vi "Actor Core.vi"(8 "error in":errorcluster, 11 "Elevator Controller in":refnum<class "Sim User Console Actor.lvclass">) -> (0 "error out":errorcluster, 3 "Actor out":refnum<class "Actor.lvclass">)   [LabVIEW 2019, in "Simulated User Console Actor.lvlib" / "Sim User Console Actor.lvclass"]
doc: "(<B>Filename</B>: Actor Framework.lvlib:Actor.lvclass:Actor Core.vi)\n\nReceives messages to the actor, reacts to them, and initiates any error handling that may shut the actor down.\n\nDescendant classes may override this VI to append parallel tasks for the actor to complete while it handles messages. Overrides use the Call Parent Method node."
uses:
  Sim User Console Actor.lvclass
  <vilib>/ActorFramework/Stop Msg/Stop Msg.lvclass
  <vilib>/ActorFramework/Actor/Actor.lvclass
  User Console Actor/User Console Actor/User Console Actor.lvclass
  C:/Workspace/CLA/Elevator AF 2nd/User Console Actor/User Console Actor/User Console Actor.lvclass
  C:/Program Files (x86)/National Instruments/LabVIEW 2019/vi.lib/ActorFramework/Actor/Actor.lvclass
  Elevator Controller/Elevator Controller Actor Messages/Restart Timing Msg/Restart Timing Msg.lvclass
  Elevator Controller/Elevator Controller Actor Messages/Change timing to seconds Msg/Change timing to seconds Msg.lvclass
  Elevator Controller/Elevator Controller Actor Messages/Set State Msg/Set State Msg.lvclass
  Elevator Controller/Elevator Controller/State -Enum.ctl
  Elevator Controller/Elevator Controller/Elevator Controller Actor.lvclass
  Elevator Controller/Elevator Controller Actor Messages/Call Emergency Msg/Call Emergency Msg.lvclass
  Door Buttons.ctl
  Elevator Call.ctl
  Floor Selection.ctl
panel:
  in  "Emergency":bool
  in  "Floor Selection":T1
  in  "Elevator Call":T2
  in  "Door Buttons":T3
  # "[Covers: UI1]\n[Covers: UI2]\n[Covers: UI2A] \n[Covers: UI2A1] \n[Covers: UI2A2] \n[Covers: UI2B] \n[Covers: UI2B1] \n[Covers: UI2B2] \n[Covers: UI2C] \n[Covers: UI2C1] \n[Covers: UI2C2] \n[Covers: UI2C3] \n[Covers: UI2D] \n[Covers: UI2D1]"
  # "Fourth Floor"
  # "Third Floor"
  # "Second Floor"
  # "First Floor"
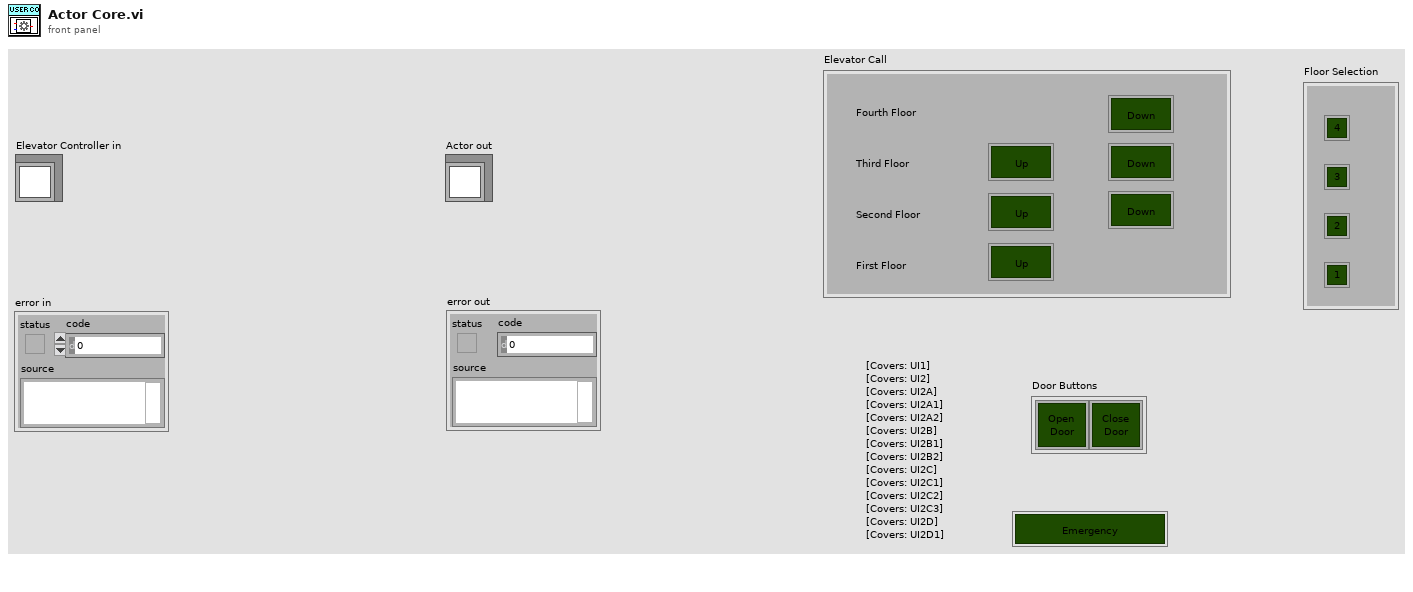
[diagram p1: front panel]
types:
  T1 = typedef "Simulated User Console Actor.lvlib/Sim User Console Actor.lvclass/Floor Selection.ctl" = cluster{"Floor4":bool, "Floor 3":bool, "Floor2":bool, "Floor1":bool}
  T2 = typedef "Simulated User Console Actor.lvlib/Sim User Console Actor.lvclass/Elevator Call.ctl" = cluster{"Up":bool, "Up 2":bool, "Up 3":bool, "Down":bool, "Down 2":bool, "Down 3":bool}
  T3 = typedef "Simulated User Console Actor.lvlib/Sim User Console Actor.lvclass/Door Buttons.ctl" = cluster{"Open Door":bool, "Close Door":bool}
  T4 = typedef "Elevator Controller Actor.lvlib/Elevator Controller Actor.lvclass/State -Enum.ctl" = enum16{"Initial", "Wait for First Request", "Start and Move", "Anaysis", "Continue Travel", "Stop at Floor", "Open and Close Door Sequence", "No Request Remaining", "Emergency Call", "Terminate Process"}
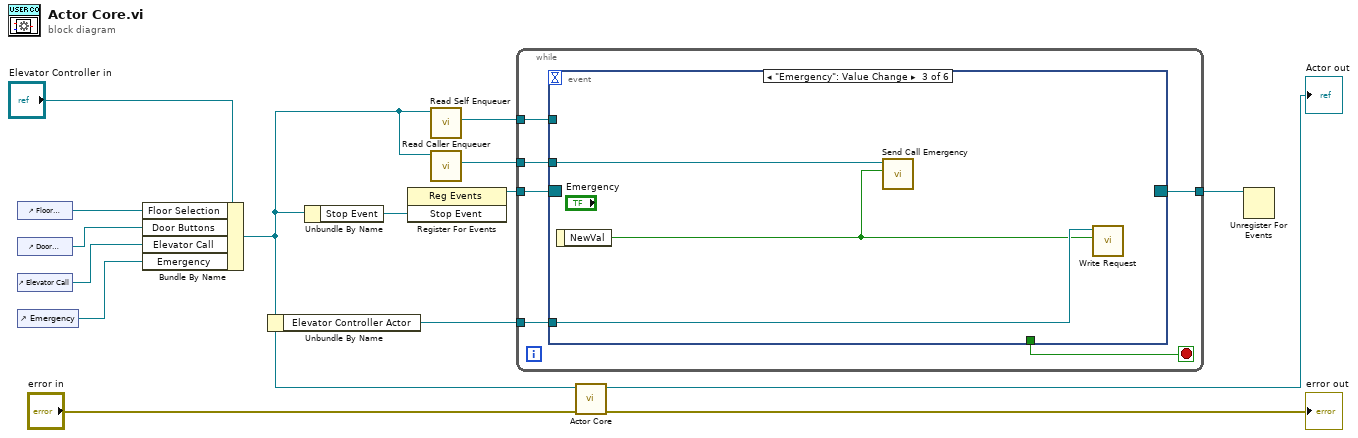
[diagram p0: block diagram]
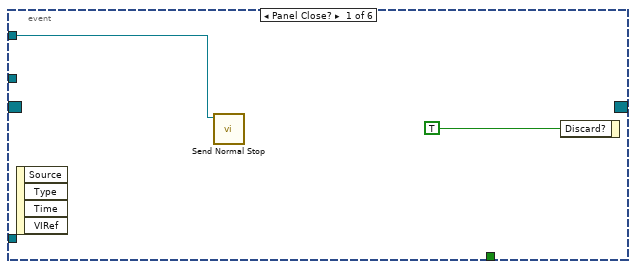
[diagram p2: hidden frame]
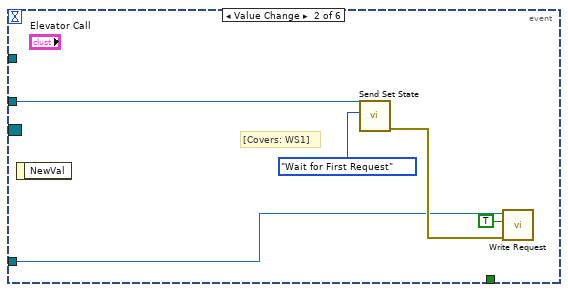
[diagram p3: hidden frame]
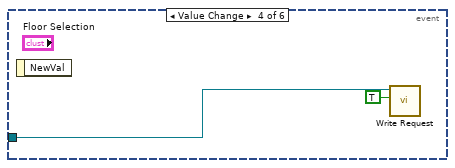
[diagram p4: hidden frame]
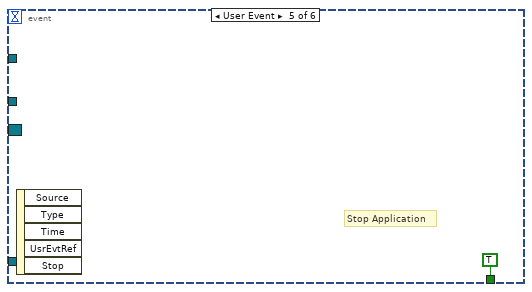
[diagram p5: hidden frame]
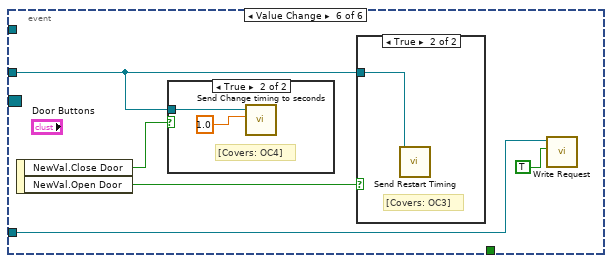
[diagram p6: hidden frame]
diagram:
  n1 = control-ref of="Floor Selection"() -> (w7:refnum<vi>)
  n2 = control-ref of="Door Buttons"() -> (w6:refnum<vi>)
  n3 = control-ref of="Elevator Call"() -> (w5:refnum<vi>)
  n4 = control-ref of="Emergency"() -> (w4:refnum<vi>)
  n5 = Bundle By Name(cluster="Elevator Controller in", "Floor Selection"=w7, "Door Buttons"=w6, "Elevator Call"=w5, "Emergency"=w4) -> (w2:refnum<class "Sim User Console Actor.lvclass">)
  n6 = Unbundle By Name(w2) -> ("Elevator Controller Actor"=w1:refnum<class "Elevator Controller Actor.lvclass">)
  n7 = Unbundle By Name(w2) -> ("Stop Event"=w12:refnum<user-event>)
  n8 = register-events(w12) -> (reference out=w11:refnum<event-registration>)  [unwired: 2 in, 1 out]
  n9 = call <vilib>:"Read Self Enqueuer.vi"("Actor"=w2) -> ("Self Enqueuer"=w9:refnum<class "Message Enqueuer.lvclass">)  [unwired: 10 in]
  n10 = call <vilib>:"Read Caller Enqueuer.vi"("Actor"=w2) -> ("Caller Enqueuer"=w3:refnum<class "Message Enqueuer.lvclass">)  [unwired: 10 in]
  n11 = while {
    tunnel: w11 -> [w20]
    tunnel: [w19] -> w10
    tunnel: w9 -> [w18]
    tunnel: w3 -> [w17]
    tunnel: w1 -> [w16]
    stop <- w21 stop-if-true
    n12 = event shown="[2] \"Emergency\": Value Change" {
      selector: w20 -> [_ _ _ _ _ _]
      dyn-events: [_ _ _ _ _ _] -> w19
      timeout: _ -> [_ _ _ _ _ _]
      tunnel: [_ _ _ _ TRUE _] -> w21
      tunnel: w18 -> [w22 _ _ _ _ _]
      tunnel: w17 -> [_ w28 w30 _ _ w37]
      tunnel: w16 -> [_ w25 w31 w33 _ w35]
      event Panel Close? {
        n13 = event-data() -> ()  [unwired: 1 in, 4 out]
        n14 = call <vilib>:"Send Normal Stop.vi"("Message Enqueuer"=w22) -> ()  [unwired: 10 in, 1 out]
        n15 = event-data("Discard?"=TRUE) -> ()  [unwired: 1 in, 1 out]
      }
      event Value Change {
        # "[Covers: WS1]"
        n16 = event-data() -> ()  [unwired: 1 in, 1 out]
        n17 = call "Send Set State.vi"("States"=State_-Enum."Wait for First Request", "Message Enqueuer"=w28) -> ("error out"=w26:errorcluster)  [unwired: 8 in, 1 out]
        n18 = call "Write Request.vi"("error in (no error)"=w26, "Request"=TRUE, "Elevator Controller Actor in"=w25) -> ()  [unwired: 7 in, 2 out]
      }
      event "Emergency": Value Change {
        n19 = event-data() -> ("NewVal"=w29:bool)  [unwired: 1 in]
        n20 = call "Send Call Emergency.vi"("Emergency"=w29, "Message Enqueuer"=w30) -> ()  [unwired: 8 in, 2 out]
        n21 = call "Write Request.vi"("Request"=w29, "Elevator Controller Actor in"=w31) -> ()  [unwired: 8 in, 2 out]
      }
      event Value Change {
        n22 = event-data() -> ()  [unwired: 1 in, 1 out]
        n23 = call "Write Request.vi"("Request"=TRUE, "Elevator Controller Actor in"=w33) -> ()  [unwired: 8 in, 2 out]
      }
      event User Event {
        # "Stop Application"
        n24 = event-data() -> ()  [unwired: 1 in, 5 out]
      }
      event Value Change {
        n25 = event-data() -> ("NewVal.Close Door"=w38:bool, "NewVal.Open Door"=w39:bool)  [unwired: 1 in]
        n26 = case shown="True" w38 {
          tunnel: w37 -> [_ w41]
          frame False {
          }
          frame True {
            # "[Covers: OC4]"
            n27 = call "Send Change timing to seconds.vi"("Time (sec)"=1.0, "Message Enqueuer"=w41) -> ()  [unwired: 8 in, 2 out]
          }
        }
        n28 = case shown="True" w39 {
          tunnel: w37 -> [_ w42]
          frame False {
          }
          frame True {
            # "[Covers: OC3]"
            n29 = call "Send Restart Timing.vi"("Message Enqueuer"=w42) -> ()  [unwired: 9 in, 2 out]
          }
        }
        n30 = call "Write Request.vi"("Request"=TRUE, "Elevator Controller Actor in"=w35) -> ()  [unwired: 8 in, 2 out]
      }
    }
  }
  n31 = call-parent "Actor Core.vi"("error in"="error in", "Actor in"=w2) -> ("error out"=→"error out":errorcluster, "Actor out"=→"Actor out":refnum<class "Actor.lvclass">)  [unwired: 8 in]
  n32 = Unregister For Events(event registration refnum=w10) -> ()  [unwired: 1 in, 1 out]
